vi "Test dropdown cell width.vi"(11 "Test Case In":refnum<class "Test Cases.lvclass">) -> (0 "error out":errorcluster, 3 "Test Case Out":refnum<class "Test Cases.lvclass">)   [LabVIEW 2024, in "Test Cases.lvclass"]
doc: "Can only be used after first StartEdit (DoubleClick) on a cell"
uses:
  Test Cases.lvclass
  C:/Program Files/National Instruments/LabVIEW 2025/vi.lib/Astemes/LUnit/Test Case.lvclass
  D:/git/Sourcegrid-LabVIEW/dll/SourceGrid.dll
  dll/SourceGrid.dll
  source/Grid/SourceGrid.lvclass
  source/Cells/Cell/Cell.lvclass
  source/Editors/Combo Box/Combo Box.lvclass
  D:/git/Sourcegrid-LabVIEW/source/Editors/Editor Base/Editor Control Base.lvclass
  <vilib>/Astemes/LUnit/Test Case.lvclass/Test Case.ctl
  <vilib>/Astemes/LUnit/Append Fail Result.vi
  <vilib>/Astemes/LUnit/Append Pass Result.vi
  <vilib>/Astemes/LUnit/Run In UI.vi
  source/Grid/Set Column Default Width.vi
  <vilib>/Astemes/LUnit/Test Case.lvclass
panel:
  in  "stop":bool
  in  "Grid Container":refnum<k24>(container)
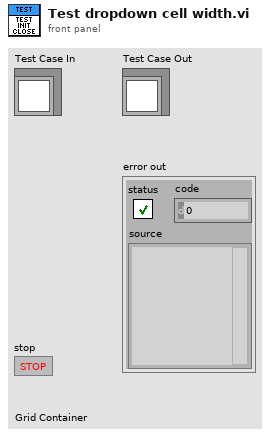
[diagram p1: front panel]
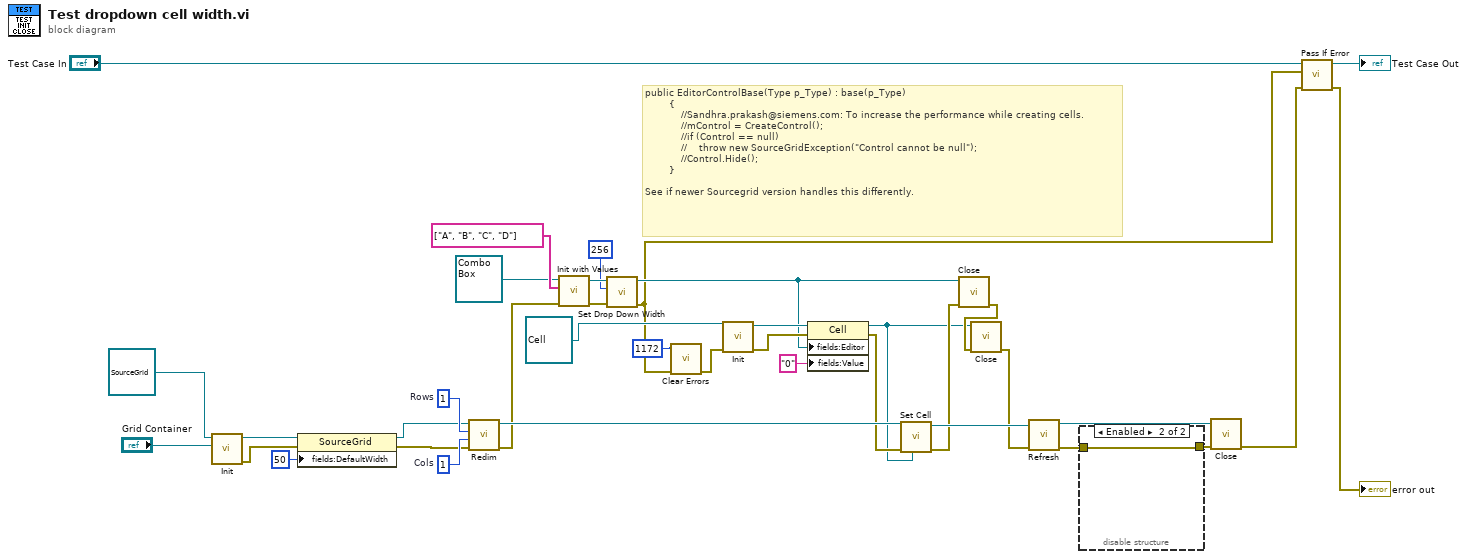
[diagram p0: block diagram]
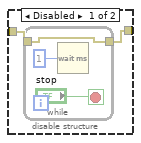
[diagram p2: hidden frame]
diagram:
  w33 = 1  # Cols
  w34 = 1  # Rows
  # "public EditorControlBase(Type p_Type) : base(p_Type)\n        {\n            //Sandhra.prakash@siemens.com: To increase the performance while creating cells.\n            //mControl = CreateControl();\n            //if (Control == null)\n            //    throw new SourceGridException(\"Control cannot be null\");\n            //Control.Hide();\n        }\n\nSee if newer Sourcegrid version handles this differently."
  n1 = call-dynamic "Init.vi"("Sourcegrid Container"="Grid Container", "Grid in"=refnum<class "SourceGrid.lvclass"> refnum) -> ("error out"=w22:errorcluster, "Grid out"=w30:refnum<class "SourceGrid.lvclass">)  [unwired: 8 in]
  n2 = property class="SourceGrid"(reference=w30, error in=w22, "fields:DefaultWidth"=50 ("DefaultWidth")) -> (reference out=w29:refnum<class "SourceGrid.lvclass">, error out=w28:errorcluster)
  n3 = call "Redim.vi"("error in"=w28, "Columns"=w33, "Rows"=w34, "Sourcegrid in"=w29) -> ("error out"=w19:errorcluster, "Sourcegrid out"=w25:refnum<class "SourceGrid.lvclass">)  [unwired: 6 in]
  n4 = call-dynamic "Init with Values.vi"("error in"=w19, "Values"=string[] ["A", "B", "C", "D"], "Combo Box in"=refnum<class "Combo Box.lvclass"> refnum ("SourceGrid.lvlib:Combo Box.lvclass")) -> ("error out"=w10:errorcluster, "Combo Box out"=w12:refnum<class "Combo Box.lvclass">)  [unwired: 7 in]
  n5 = call "Set Drop Down Width.vi"("error in"=w10, "Drop Down Width"=256, "Combo Box in"=w12) -> ("error out"=w4:errorcluster, "Combo Box out"=w8:refnum<class "Combo Box.lvclass">)  [unwired: 7 in]
  n6 = call <vilib>:"Clear Errors.vi"("error in (no error)"=w4, "specific error code to clear (0: all)"=1172) -> ("error out"=w3:errorcluster)  [unwired: 4 in, 1 out]
  n7 = call-dynamic "Init.vi"("error in"=w3, "Cell in"=refnum<class "Cell.lvclass"> refnum) -> ("error out"=w16:errorcluster, "Cell out"=w17:refnum<class "Cell.lvclass">)  [unwired: 8 in]
  n8 = property class="Cell"(reference=w17, error in=w16, "fields:Editor"=w8, "fields:Value"="0") -> (reference out=w1:refnum<class "Cell.lvclass">, error out=w18:errorcluster)
  n9 = call "Set Cell.vi"("Cell"=w1, "error in"=w18, "Sourcegrid in"=w25) -> ("error out"=w7:errorcluster, "Sourcegrid out"=w26:refnum<class "SourceGrid.lvclass">)  [unwired: 7 in]
  n10 = call-dynamic "Close.vi"("error in"=w7, "Combo Box in"=w8) -> ("error out"=w6:errorcluster)  [unwired: 8 in, 1 out]
  n11 = call-dynamic "Close.vi"("error in"=w6, "Cell in"=w1) -> ("error out"=w5:errorcluster)  [unwired: 8 in, 1 out]
  n12 = call "Refresh.vi"("error in"=w5, "SourceGrid in"=w26) -> ("error out"=w13:errorcluster, "SourceGrid out"=w23:refnum<class "SourceGrid.lvclass">)  [unwired: 8 in]
  n13 = disable-structure shown="Enabled" {
    disable-tunnel: w13 -> [w39 w43]
    disable-tunnel: [w38 w43] -> w9
    frame Disabled {
      n14 = while {
        tunnel: w39 -> [w40]
        tunnel: [w40] -> w38
        stop <- "stop" stop-if-true
        n15 = Wait (ms)(milliseconds to wait=u32 1) -> ()  [unwired: 1 out]
      }
    }
    frame Enabled {
    }
  }
  n16 = call-dynamic "Close.vi"("error in"=w9, "Sourcegrid in"=w23) -> ("error out"=w32:errorcluster)  [unwired: 8 in, 1 out]
  n17 = call <vilib>:"Pass If Error.vi"("error in (no error)"=w32, "Assert error"=w4, "LUnit Test Case In"="Test Case In") -> ("error out"=→"error out":errorcluster, "LUnit Test Case Out"=→"Test Case Out":refnum<class "Test Cases.lvclass">)  [unwired: 7 in]
